vi "Populate Response Core.vi"(8 "error in (no error)":errorcluster, 10 "Timeout if waiting(-1ms)":i32=-1, 11 "Send Function":T1) -> (0 "error out":errorcluster, 3 "Response Core":refnum<class "Response Core.lvclass">)   [LabVIEW 2020, in "Publisher.lvlib" / "Response Msg.lvclass"]
uses:
  Response Msg.lvclass
  Response Core/Controls/Ctl_SendFunction.ctl
  Response Core/Response Core/Response Core.lvclass
  Response Core/Send and Forget Core/Send and Forget Core.lvclass
  C:/Current projects/WS/Framework/Framework/Actors/Publisher/Messages/Response Msg/Response Core/Response Core/Response Core.lvclass
  Response Core/Request Reply Core/Request Reply Core.lvclass
  Response Core/Interruptible Reply Core/Interruptible Reply Core.lvclass/Interruptible Reply Core.ctl
  Response Core/Interruptible Reply Core/Interruptible Reply Core.lvclass
  Publisher.lvlib
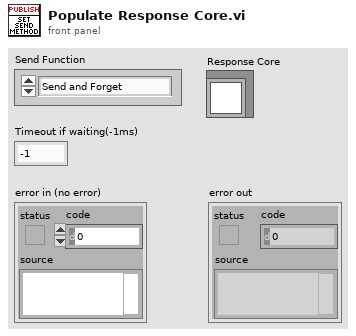
[diagram p1: front panel]
types:
  T1 = typedef "Publisher.lvlib/Ctl_SendFunction.ctl" = enum16{"Send and Forget", "Request Reply", "Await Reply"}
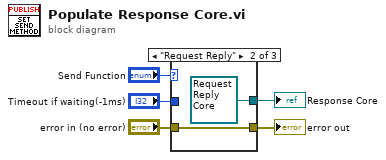
[diagram p0: block diagram]
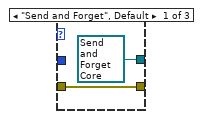
[diagram p2: hidden frame]
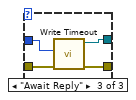
[diagram p3: hidden frame]
diagram:
  n1 = case shown="\"Request Reply\"" "Send Function" {
    tunnel: [refnum<class "Send and Forget Core.lvclass"> refnum ("Publisher.lvlib:Send and Forget Core.lvclass") refnum<class "Request Reply Core.lvclass"> refnum ("Publisher.lvlib:Request Reply Core.lvclass") w12] -> w4
    tunnel: "Timeout if waiting(-1ms)" -> [_ _ w13]
    tunnel: "error in (no error)" -> [w7 w8 w11]
    tunnel: [w7 w8 w10] -> w1
    frame "Send and Forget", Default {
    }
    frame "Request Reply" {
    }
    frame "Await Reply" {
      n2 = call "Write Timeout.vi"("error in (no error)"=w11, "Timeout time(-1ms)"=w13) -> ("error out"=w10:errorcluster, "Interruptible Reply Core out"=w12:refnum<class "Interruptible Reply Core.lvclass">)  [unwired: 8 in]
    }
  }
  "error out" <- w1
  "Response Core" <- w4
